vi "Add to Project.vi"(8 "error in (no error)":errorcluster, 11 "Coupled Message Scripter in":refnum<class "Coupled Message Scripter.lvclass">) -> (0 "error out":errorcluster, 3 "Coupled Message Scripter out":refnum<class "Coupled Message Scripter.lvclass">)   [LabVIEW 2020, in "Message Maker.lvlib" / "Coupled Message Scripter.lvclass"]
uses:
  Coupled Message Scripter.lvclass
  Message Maker.lvlib
  Message Scripter/Message Scripter.lvclass
  _support/Localized Strings.vi
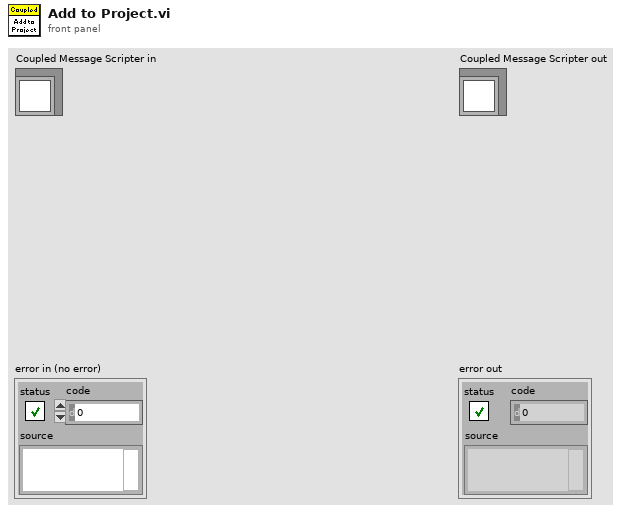
[diagram p1: front panel]
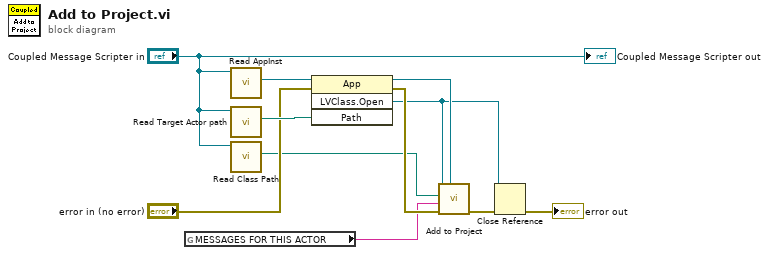
[diagram p0: block diagram]
diagram:
  n1 = global read "Localized Strings.vi" "MESSAGES FOR THIS ACTOR"() -> (w1:string)
  n2 = call "Read AppInst.vi"("Message Maker in"="Coupled Message Scripter in") -> ("AppInst"=w3:refnum<vi>)  [unwired: 10 in]
  n3 = call "Read Target Actor path.vi"("Message Scripter in"="Coupled Message Scripter in") -> ("Target Actor path"=w11:path)  [unwired: 10 in]
  n4 = call "Read Class Path.vi"("Message Scripter in"="Coupled Message Scripter in") -> ("Class Path"=w4:path)  [unwired: 10 in]
  n5 = invoke class="App" method="LVClass.Open"(reference=w3, error in="error in (no error)", "Path"=w11) -> (reference out=w10:refnum<vi>, error out=w8:errorcluster, "LVClass.Open"=w5:refnum<vi>)  [unwired: 1 in, 1 out]
  n6 = call "Add to Project.vi"("AppInst"=w10, "error in (no error)"=w8, "Folder"=w1, "Class Path"=w4, "Actor"=w5) -> ("error out"=w7:errorcluster)  [unwired: 6 in]
  n7 = Close Reference(reference=w5, error in (no error)=w7) -> (error out=→"error out":errorcluster)
  "Coupled Message Scripter out" <- "Coupled Message Scripter in"
